vi "pot voltage to angle.vi"(0 "AIDeviceRef":T1) -> (1 "Average Angle":dbl, 2 "Angle":dbl, 3 "Adjusted Angle":dbl)   [LabVIEW 2012]
uses:
  <vilib>/Rock Robotics/WPI/AnalogChannel/WPI_AnalogChannelDevRef.ctl
  <vilib>/Rock Robotics/SystemInterfaces/Typedef/FPGA_TypedefAnalogModule.ctl
  <vilib>/Rock Robotics/SystemInterfaces/AI/FPGA_AIChannel.ctl
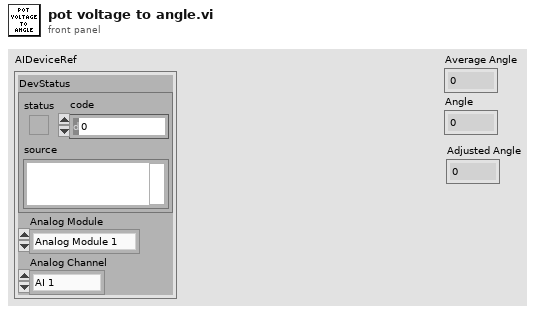
[diagram p1: front panel]
types:
  T1 = typedef "WPI_AnalogChannelDevRef.ctl" = cluster{"DevStatus":errorcluster, "Analog Module":T2, "Analog Channel":T3}
  T2 = typedef "FPGA_TypedefAnalogModule.ctl" = enum16{"Analog Module 1", "Analog Module 2"}
  T3 = typedef "FPGA_AIChannel.ctl" = enum8{"AI 1", "AI 2", "AI 3", "AI 4", "AI 5", "AI 6", "AI 7", "AI 8", "Invalid"}
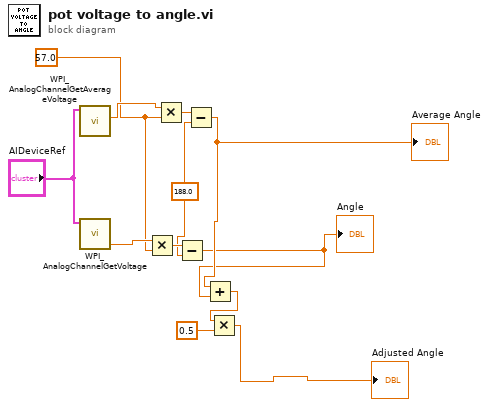
[diagram p0: block diagram]
diagram:
  w2 = 188.0 ("-")
  w3 = 57.0 ("X")
  n1 = call <vilib>:"WPI_AnalogChannelGetAverageVoltage.vi"("AIDeviceRef"="AIDeviceRef") -> ("Voltage"=w12:dbl)  [unwired: 8 in, 2 out]
  n2 = call <vilib>:"WPI_AnalogChannelGetVoltage.vi"("AIDeviceRef"="AIDeviceRef") -> ("Voltage"=w9:dbl)  [unwired: 8 in, 2 out]
  n3 = Multiply(x=w9, y=w3) -> (x*y=w10:dbl)
  n4 = Multiply(x=w12, y=w3) -> (x*y=w11:dbl)
  n5 = Subtract(x=w10, y=w2) -> (x-y=w6:dbl)
  "Angle" <- w6
  n6 = Subtract(x=w11, y=w2) -> (x-y=w7:dbl)
  "Average Angle" <- w7
  n7 = Add(x=w7, y=w6) -> (x+y=w5:dbl)
  n8 = Multiply(x=w5, y=0.5) -> (x*y=→"Adjusted Angle":dbl)
